vi "ACPV2_Remotecontrol.vi"() -> ()   [LabVIEW 2016]
uses:
  <vilib>/Instr/_visa.llb/VISA Configure Serial Port (Instr).vi
panel:
  in  "Set time (us)":dbl=50.0 min=0.0 max=400.0
  in  "Set time":bool
  in  "Set valve":bool
  out "Voltage":string="200V"
  out "Time":string="50us"
  out "Current mode":string=" LOCAL"
  out "Firmware":string="1.1.2_200"
  in  "Set mode":bool
  in  "stop":bool
  # "Piezo valve control panel"
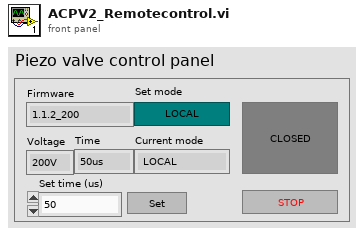
[diagram p1: front panel]
types:
  T1 = enum8{"Enabled", "Disabled", "Disabled and Grayed Out"}
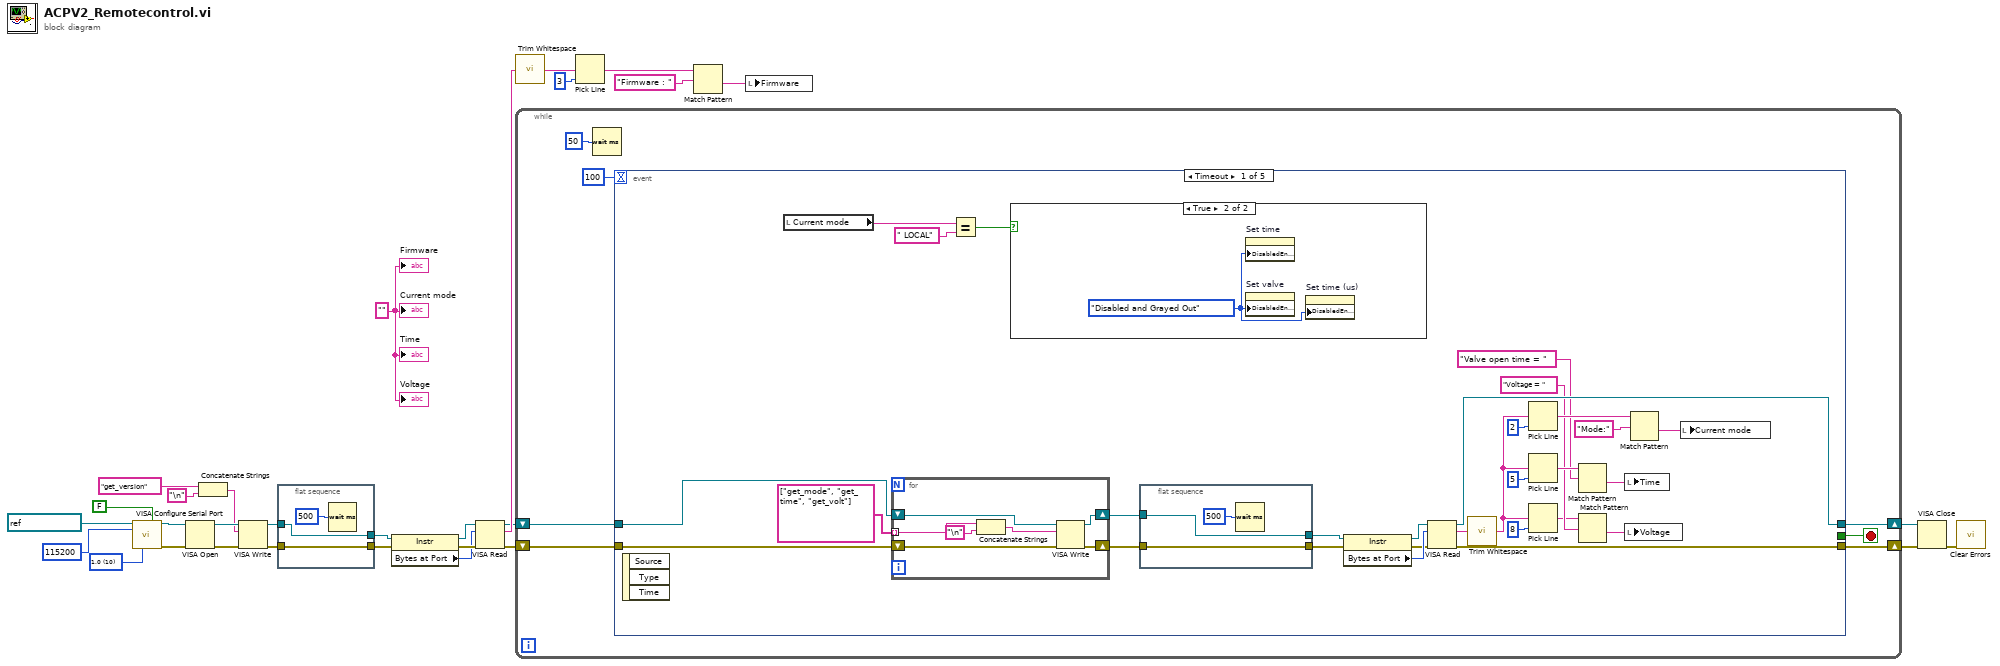
[diagram p0: block diagram]
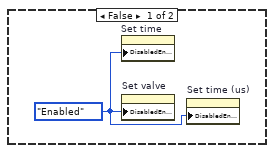
[diagram p2: hidden frame]
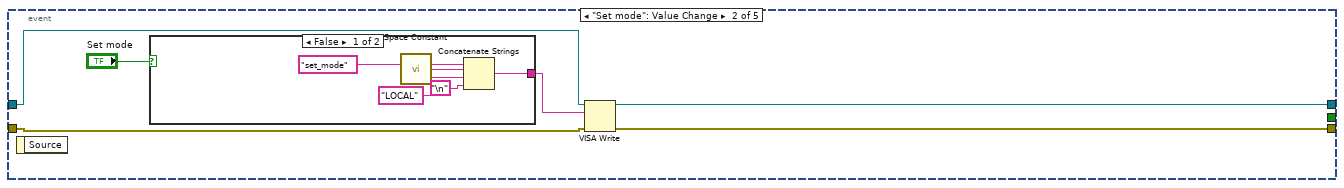
[diagram p3: hidden frame]
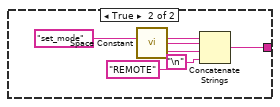
[diagram p4: hidden frame]
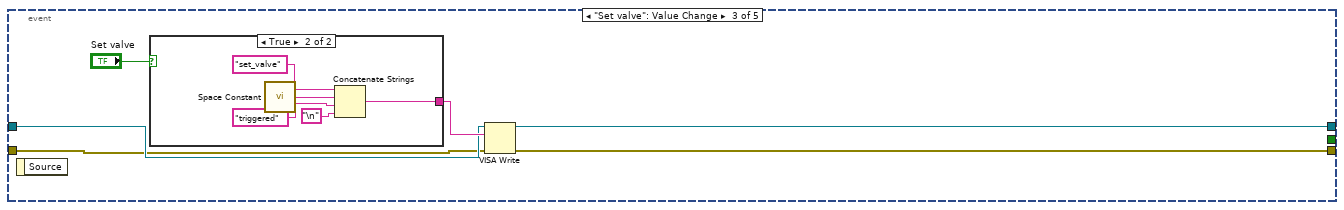
[diagram p5: hidden frame]
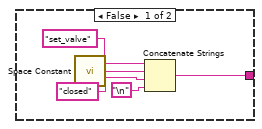
[diagram p6: hidden frame]
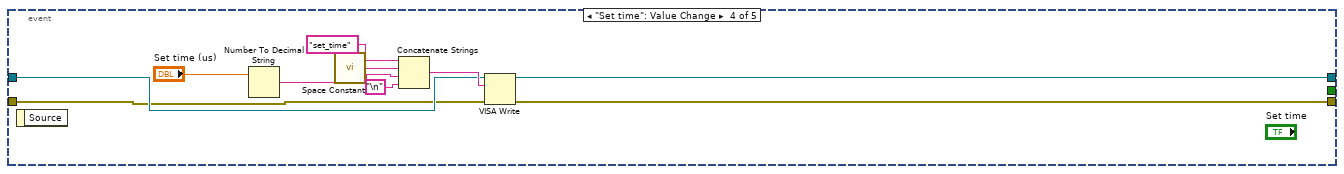
[diagram p7: hidden frame]
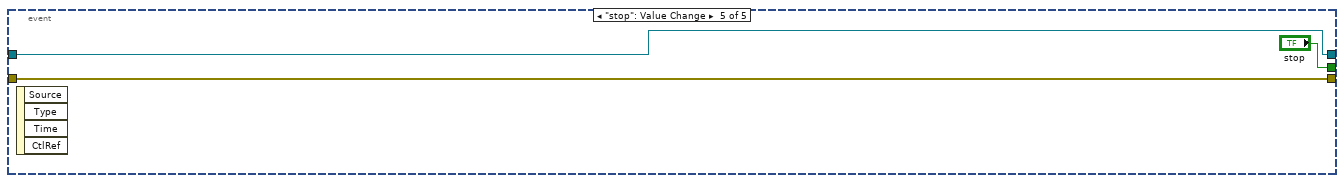
[diagram p8: hidden frame]
diagram:
  w29 = u16 10 items=["1.0"=10, "1.5"=15, "2.0"=20] ("stop bits (10: 1 bit)")
  w1 = "" ("Firmware")
  n1 = call-poly "VISA Configure Serial Port"("VISA resource name"=refnum<visa-resource-name> "COM3", "Enable Termination\nChar (T)"=FALSE ("Enable Termination\nChar (T)"), "baud rate (9600)"=u32 115200, "stop bits (10: 1 bit)"=w29) -> ("VISA resource name out"=w15:refnum<visa-resource-name>, "error out"=w11:errorcluster)  [unwired: 10 in]
  n2 = VISA Open(error in (no error)=w11, VISA resource name=w15) -> (VISA resource name=w20:refnum<visa-resource-name>, error out=w21:errorcluster)  [unwired: 3 in]
  n3 = Concatenate Strings("get_version" ("string"), "\n") -> (w19:string)
  n4 = VISA Write(VISA resource name=w20, write buffer=w19, error in (no error)=w21) -> (VISA resource name out=w10:refnum<visa-resource-name>, error out=w9:errorcluster)  [unwired: 1 out]
  n5 = flat-sequence {
    tunnel: [w33] -> w8
    tunnel: w10 -> [w33]
    tunnel: w9 -> [w32]
    tunnel: [w32] -> w7
    frame #0 {
      n6 = Wait (ms)(milliseconds to wait=u32 500) -> ()  [unwired: 1 out]
    }
  }
  n7 = property class="Instr"(reference=w8, error in=w7) -> (reference out=w6:refnum<visa-resource-name>, error out=w5:errorcluster, "Bytes at Port"=w4:u32)
  n8 = VISA Read(VISA resource name=w6, byte count=w4, error in (no error)=w5) -> (VISA resource name out=w13:refnum<visa-resource-name>, read buffer=w26:string, error out=w3:errorcluster)  [unwired: 1 out]
  n9 = call <vilib>:"Trim Whitespace.vi"("string"=w26) -> ("trimmed string"=w22:string)  [unwired: 1 in]
  n10 = while {
    shift-right: [w40] -> w12
    shift-left: w13 -> [w37]
    shift-right: [w35] -> w2
    shift-left: w3 -> [w36]
    stop <- w38 stop-if-true
    n11 = Wait (ms)(milliseconds to wait=u32 50) -> ()  [unwired: 1 out]
    n12 = event shown="[0] Timeout" {
      selector: _ -> [_ _ _ _ _]
      dyn-events: _ -> [_ _ _ _ _]
      timeout: 100 -> [_ _ _ _ _]
      tunnel: [w60 w85 w101 w122 w125] -> w40
      tunnel: [_ _ _ _ "stop"] -> w38
      tunnel: w37 -> [w62 w84 w100 w121 w125]
      tunnel: w36 -> [w61 w83 w99 w120 w124]
      tunnel: [w59 w82 w98 w119 w124] -> w35
      event Timeout {
        n13 = event-data() -> ()  [unwired: 1 in, 3 out]
        n14 = local read "Current mode"() -> (w43:string)
        n15 = for {
          shift-right: [w78] -> w69
          shift-left: w62 -> [w76]
          shift-right: [w77] -> w68
          shift-left: w61 -> [w75]
          tunnel: string[] ["get_mode", "get_time", "get_volt"] -> [w72] mode=indexing
          n16 = Concatenate Strings(w72, "\n") -> (w73:string)
          n17 = VISA Write(VISA resource name=w76, write buffer=w73, error in (no error)=w75) -> (VISA resource name out=w78:refnum<visa-resource-name>, error out=w77:errorcluster)  [unwired: 1 out]
        }
        n18 = Equal?(x=w43, y=" LOCAL") -> (x = y?=w41:bool)
        n19 = case shown="True" w41 {
          frame False {
            w70 = T1."Enabled" ("Disabled")
            n20 = property on="Set time" class="Bool"("DisabledEnum"=w70) -> ()  [unwired: 2 in, 2 out]
            n21 = property on="Set valve" class="Bool (strict)"("DisabledEnum"=w70) -> ()  [unwired: 2 in, 2 out]
            n22 = property on="Set time (us)" class="DigNum (strict)"("DisabledEnum"=w70) -> ()  [unwired: 2 in, 2 out]
          }
          frame True {
            w71 = T1."Disabled and Grayed Out" ("Disabled")
            n23 = property on="Set time" class="Bool"("DisabledEnum"=w71) -> ()  [unwired: 2 in, 2 out]
            n24 = property on="Set valve" class="Bool (strict)"("DisabledEnum"=w71) -> ()  [unwired: 2 in, 2 out]
            n25 = property on="Set time (us)" class="DigNum (strict)"("DisabledEnum"=w71) -> ()  [unwired: 2 in, 2 out]
          }
        }
        n26 = flat-sequence {
          tunnel: [w81] -> w67
          tunnel: w69 -> [w81]
          tunnel: w68 -> [w80]
          tunnel: [w80] -> w66
          frame #0 {
            n27 = Wait (ms)(milliseconds to wait=u32 500) -> ()  [unwired: 1 out]
          }
        }
        n28 = property class="Instr"(reference=w67, error in=w66) -> (reference out=w65:refnum<visa-resource-name>, error out=w63:errorcluster, "Bytes at Port"=w64:u32)
        n29 = VISA Read(VISA resource name=w65, byte count=w64, error in (no error)=w63) -> (VISA resource name out=w60:refnum<visa-resource-name>, read buffer=w55:string, error out=w59:errorcluster)  [unwired: 1 out]
        n30 = call <vilib>:"Trim Whitespace.vi"("string"=w55) -> ("trimmed string"=w45:string)  [unwired: 1 in]
        n31 = Pick Line(multi-line string=w45, line index=2) -> (output string=w56:string)  [unwired: 1 in]
        n32 = Pick Line(multi-line string=w45, line index=5) -> (output string=w52:string)  [unwired: 1 in]
        n33 = Pick Line(multi-line string=w45, line index=8) -> (output string=w49:string)  [unwired: 1 in]
        n34 = Match Pattern(string=w52, regular expression="Valve open time = ") -> (after substring=w48:string)  [unwired: 1 in, 3 out]
        n35 = Match Pattern(string=w49, regular expression="Voltage = ") -> (after substring=w47:string)  [unwired: 1 in, 3 out]
        n36 = local write "Time"(w48) -> ()
        n37 = local write "Voltage"(w47) -> ()
        n38 = Match Pattern(string=w56, regular expression="Mode:") -> (after substring=w58:string)  [unwired: 1 in, 3 out]
        n39 = local write "Current mode"(w58) -> ()
      }
      event "Set mode": Value Change {
        n40 = event-data() -> ()  [unwired: 1 in, 1 out]
        n41 = case shown="False" "Set mode" {
          tunnel: [w88 w93] -> w86
          frame False {
            n42 = call <vilib>:"Space Constant.vi"() -> ("String"=w90:string)
            n43 = Concatenate Strings("set_mode" ("string"), w90, "LOCAL" ("string"), "\n") -> (w88:string)
          }
          frame True {
            n44 = call <vilib>:"Space Constant.vi"() -> ("String"=w95:string)
            n45 = Concatenate Strings("set_mode" ("string"), w95, "REMOTE" ("string"), "\n") -> (w93:string)
          }
        }
        n46 = VISA Write(VISA resource name=w84, write buffer=w86, error in (no error)=w83) -> (VISA resource name out=w85:refnum<visa-resource-name>, error out=w82:errorcluster)  [unwired: 1 out]
      }
      event "Set valve": Value Change {
        n47 = event-data() -> ()  [unwired: 1 in, 1 out]
        n48 = case shown="True" "Set valve" {
          tunnel: [w104 w109] -> w102
          frame False {
            n49 = call <vilib>:"Space Constant.vi"() -> ("String"=w106:string)
            n50 = Concatenate Strings("set_valve" ("string"), w106, "closed" ("string"), "\n") -> (w104:string)
          }
          frame True {
            n51 = call <vilib>:"Space Constant.vi"() -> ("String"=w111:string)
            n52 = Concatenate Strings("set_valve" ("string"), w111, "triggered" ("string"), "\n") -> (w109:string)
          }
        }
        n53 = VISA Write(VISA resource name=w100, write buffer=w102, error in (no error)=w99) -> (VISA resource name out=w101:refnum<visa-resource-name>, error out=w98:errorcluster)  [unwired: 1 out]
      }
      event "Set time": Value Change {
        n54 = event-data() -> ()  [unwired: 1 in, 1 out]
        n55 = Number To Decimal String(number="Set time (us)") -> (decimal integer string=w114:string)  [unwired: 1 in]
        n56 = call <vilib>:"Space Constant.vi"() -> ("String"=w117:string)
        n57 = Concatenate Strings("set_time" ("string"), w117, w114, "\n") -> (w123:string)
        n58 = VISA Write(VISA resource name=w121, write buffer=w123, error in (no error)=w120) -> (VISA resource name out=w122:refnum<visa-resource-name>, error out=w119:errorcluster)  [unwired: 1 out]
      }
      event "stop": Value Change {
        n59 = event-data() -> ()  [unwired: 1 in, 4 out]
      }
    }
  }
  n60 = Pick Line(multi-line string=w22, line index=3) -> (output string=w23:string)  [unwired: 1 in]
  n61 = Match Pattern(string=w23, regular expression="Firmware : ") -> (after substring=w28:string)  [unwired: 1 in, 3 out]
  n62 = local write "Firmware"(w28) -> ()
  n63 = VISA Close(VISA resource name=w12, error in (no error)=w2) -> (error out=w30:errorcluster)
  n64 = call <vilib>:"Clear Errors.vi"("error in (no error)"=w30) -> ()  [unwired: 5 in, 2 out]
  "Firmware" <- w1
  "Current mode" <- w1
  "Time" <- w1
  "Voltage" <- w1
